vi "SetDictionary.vi"(8 "error in (no error)":errorcluster caption="Fehler (Eingang, kein Fehler)", 10 "LvDictionary.lvlib:DictionaryString.lvclass":refnum<class "DictionaryString.lvclass">, 11 "PassDataAround Eingang":refnum<class "PassDataAround.lvclass"> caption="DNL_LabVIEW Object in") -> (0 "error out":errorcluster caption="Fehler (Ausgang)", 3 "PassDataAround Ausgang":refnum<class "PassDataAround.lvclass"> caption="DNL_LabVIEW Object out")   [LabVIEW 2013, in "PassDataAround.lvlib" / "PassDataAround.lvclass"]
uses:
  PassDataAround.lvclass
  LvDictionary/DictionaryStringClass/DictionaryString.lvclass
  PassDataAround.lvclass/PassDataAround.ctl
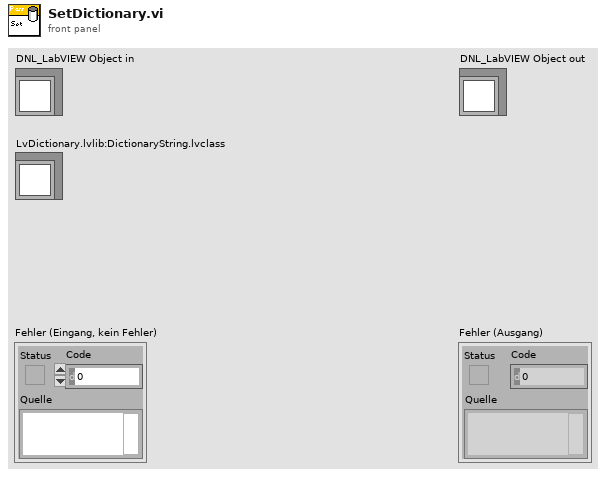
[diagram p1: front panel]
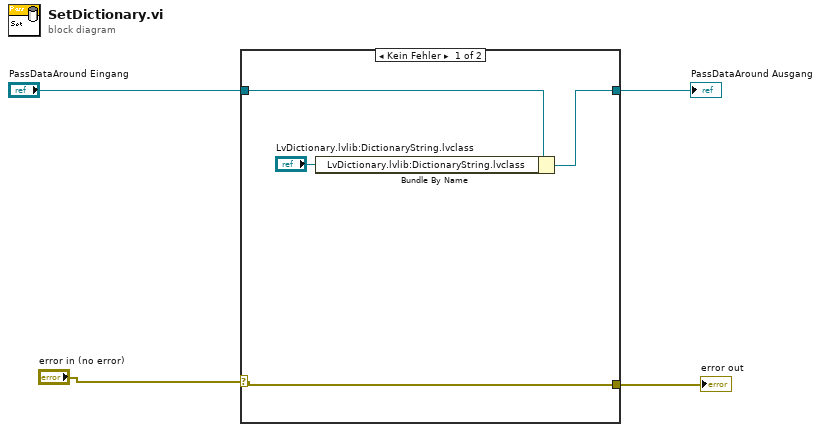
[diagram p0: block diagram]
diagram:
  n1 = case shown="Kein Fehler" "error in (no error)" {
    selector: "error in (no error)" -> [w8 w10]
    tunnel: [w8 w10] -> w3
    tunnel: "PassDataAround Eingang" -> [w7 w9]
    tunnel: [w6 w9] -> w2
    frame No Error {
      n2 = Bundle By Name(cluster=w7, "LvDictionary.lvlib:DictionaryString.lvclass"="LvDictionary.lvlib:DictionaryString.lvclass") -> (w6:refnum<class "PassDataAround.lvclass">)
    }
    frame Error {
    }
  }
  "error out" <- w3
  "PassDataAround Ausgang" <- w2
